vi "Create Message Setter (from Accessor).vi"(8 "error in (no error)":errorcluster, 10 "RPC Message Name":string, 11 "RPC Messages Folder (ProjectItem) in":refnum<vi>) -> (0 "error out":errorcluster, 1 "Created ?":bool, 2 "Getter VI out":refnum<vi>, 3 "RPC Messages Folder (ProjectItem) out":refnum<vi>)   [LabVIEW 2019, in "gRPC Template Creation Utility.lvlib"]
uses:
  gRPC Template Creation Utility.lvlib
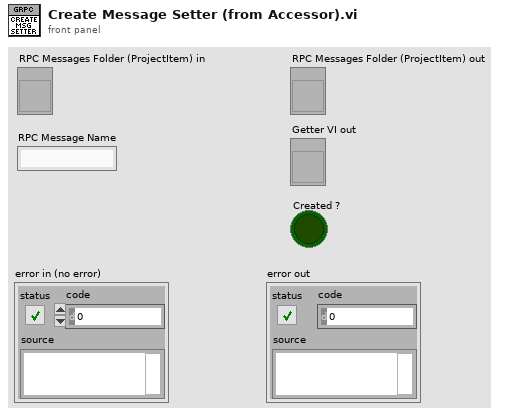
[diagram p1: front panel]
types:
  T1 = enum32{"invalid VI type", "Standard VI", "Control VI", "Global VI", "Polymorphic VI", "Configuration VI", "SubSystem", "Facade VI", "Method VI"}
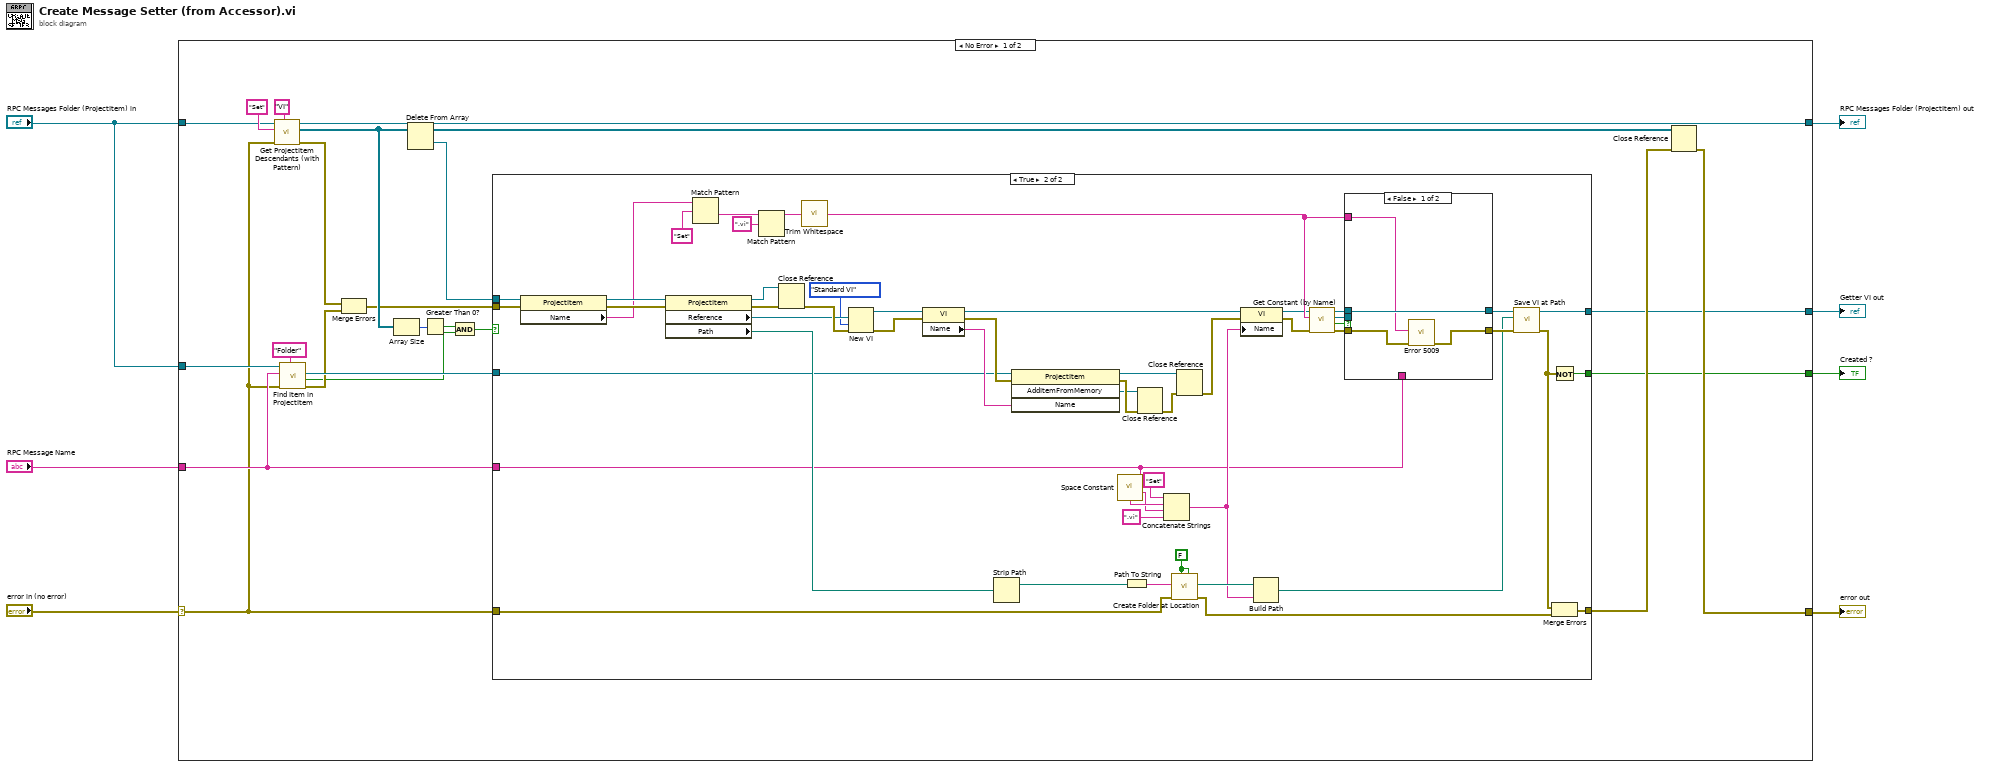
[diagram p0: block diagram]
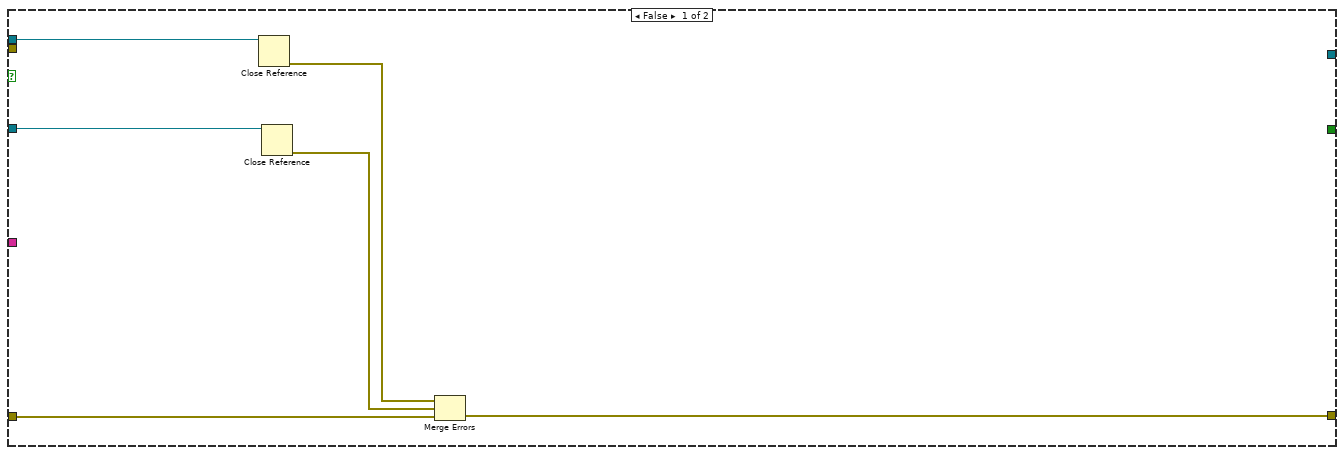
[diagram p2: hidden frame]
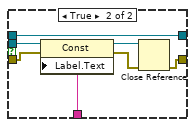
[diagram p3: hidden frame]
diagram:
  n1 = case shown="No Error" "error in (no error)" {
    selector: "error in (no error)" -> [w13 w100]
    tunnel: "RPC Message Name" -> [w25 _]
    tunnel: "RPC Messages Folder (ProjectItem) in" -> [w23 _]
    tunnel: "RPC Messages Folder (ProjectItem) in" -> [w18 w99]
    tunnel: [w11 w100] -> w4
    tunnel: [w10 w99] -> w3
    tunnel: [w9 _] -> w2
    tunnel: [w8 _] -> w1
    frame No Error {
      n2 = call "Get ProjectItem Descendants (with Pattern).vi"("Type"="VI", "error in (no error)"=w13, "Pattern"="Set", "ProjectItem in"=w18) -> ("error out"=w17:errorcluster, "ProjectItem descendents"=w24:refnum<vi>[], "ProjectItem out"=w10:refnum<vi>)  [unwired: 5 in]
      n3 = call "Find Item in ProjectItem.vi"("Item Type"="Folder", "error in (no error)"=w13, "Name"=w25, "ProjectItem in"=w23) -> ("error out"=w16:errorcluster, "Found ?"=w15:bool, "Item Refnum out"=w21:refnum<vi>)  [unwired: 4 in, 1 out]
      n4 = Merge Errors(w17, w16) -> (w14:errorcluster)
      n5 = Array Size(array=w24) -> (size(s)=w22:i32)
      n6 = Delete From Array(array=w24) -> (deleted portion=w27:refnum<vi>, array with subset deleted=w30:refnum<vi>[])  [unwired: 2 in]
      n7 = Greater Than 0?(x=w22) -> (x > 0?=w20:bool)
      n8 = And(x=w20, y=w15) -> (x .and. y?=w19:bool)
      n9 = case shown="True" w19 {
        tunnel: w25 -> [_ w38]
        tunnel: [w33 w84] -> w12
        tunnel: [_ w45] -> w8
        tunnel: w27 -> [w36 w59]
        tunnel: [_ w69] -> w9
        tunnel: w21 -> [w31 w64]
        tunnel: w13 -> [w32 w63]
        tunnel: w14 -> [_ w58]
        frame False {
          n10 = Close Reference(reference=w36) -> (error out=w34:errorcluster)  [unwired: 1 in]
          n11 = Close Reference(reference=w31) -> (error out=w35:errorcluster)  [unwired: 1 in]
          n12 = Merge Errors(w34, w35, w32) -> (w33:errorcluster)
        }
        frame True {
          w82 = FALSE ("Use Relative (F)")
          n13 = property class="ProjectItem"(reference=w59, error in=w58) -> (reference out=w57:refnum<vi>, error out=w56:errorcluster, "Name"=w55:string)
          n14 = property class="ProjectItem"(reference=w57, error in=w56) -> (reference out=w87:refnum<vi>, error out=w85:errorcluster, "Reference"=w75:refnum<vi>, "Path"=w78:path)
          n15 = Match Pattern(string=w55, regular expression="Set") -> (after substring=w53:string)  [unwired: 1 in, 3 out]
          n16 = Match Pattern(string=w53, regular expression=".vi") -> (before substring=w42:string)  [unwired: 1 in, 3 out]
          n17 = Close Reference(reference=w87, error in (no error)=w85) -> (error out=w86:errorcluster)
          n18 = call <vilib>:"Trim Whitespace.vi"("string"=w42) -> ("trimmed string"=w51:string)  [unwired: 1 in]
          n19 = New VI(8:w86, 9:T1."Standard VI" ("vi type (standard vi)"), 10:w75) -> (0:w74:errorcluster, 3:w72:refnum<vi>)  [unwired: 1 in, 3 out]
          n20 = property class="VI"(reference=w72, error in=w74) -> (reference out=w79:refnum<vi>, error out=w80:errorcluster, "Name"=w76:string)
          n21 = Strip Path(path=w78) -> (stripped path=w37:path)  [unwired: 1 out]
          n22 = invoke class="ProjectItem" method="AddItemFromMemory"(reference=w64, error in=w80, "Name"=w76) -> (reference out=w71:refnum<vi>, error out=w62:errorcluster, "AddItemFromMemory"=w61:refnum<vi>)  [unwired: 1 in, 1 out]
          n23 = call <vilib>:"Space Constant.vi"() -> ("String"=w67:string)
          n24 = Path To String(path=w37) -> (string=w77:string)
          n25 = Close Reference(reference=w61, error in (no error)=w62) -> (error out=w60:errorcluster)
          n26 = Concatenate Strings("Set" ("string"), w67, w38, ".vi" ("string")) -> (w65:string)
          n27 = call "Create Folder at Location.vi"("Override existing (F)"=w82, "Use Relative (F)"=w82, "Error In"=w63, "Path"=w77) -> ("Error Out"=w83:errorcluster, "Full path out"=w81:path)  [unwired: 5 in, 1 out]
          n28 = Close Reference(reference=w71, error in (no error)=w60) -> (error out=w70:errorcluster)
          n29 = property class="VI"(reference=w79, error in=w70, "Name"=w65) -> (reference out=w49:refnum<vi>, error out=w48:errorcluster)
          n30 = Build Path(base path=w81, name or relative path=w65) -> (appended path=w44:path)
          n31 = call "Get Constant (by Name).vi"("error in (no error)"=w48, "Constant Label"=w51, "Owner VI in"=w49) -> ("error out"=w47:errorcluster, "Found ?"=w41:bool, "Const ref out"=w50:refnum<vi>, "Owner VI out"=w40:refnum<vi>)  [unwired: 5 in]
          n32 = case shown="False" w41 {
            tunnel: w50 -> [_ w98]
            tunnel: w38 -> [_ w97]
            tunnel: w47 -> [w90 w96]
            tunnel: [w89 w93] -> w46
            tunnel: w40 -> [w91 w92]
            tunnel: [w91 w92] -> w39
            tunnel: w51 -> [w88 _]
            frame False {
              n33 = call "Error 5009.vi"("error in (no error)"=w90, "Cluster Definition Constant"=w88) -> ("error out"=w89:errorcluster)  [unwired: 9 in]
            }
            frame True {
              n34 = property class="Const"(reference=w98, error in=w96, "Label.Text"=w97) -> (reference out=w95:refnum<vi>, error out=w94:errorcluster)
              n35 = Close Reference(reference=w95, error in (no error)=w94) -> (error out=w93:errorcluster)
            }
          }
          n36 = call "Save VI at Path.vi"("error in (no error)"=w46, "Path"=w44, "VI in"=w39) -> ("error out"=w43:errorcluster, "VI out"=w45:refnum<vi>)  [unwired: 6 in, 1 out]
          n37 = Not(x=w43) -> (.not. x?=w69:bool)
          n38 = Merge Errors(w43, w83) -> (w84:errorcluster)
        }
      }
      n39 = Close Reference(reference=w30, error in (no error)=w12) -> (error out=w11:errorcluster)
    }
    frame Error {
    }
  }
  "error out" <- w4
  "RPC Messages Folder (ProjectItem) out" <- w3
  "Created ?" <- w2
  "Getter VI out" <- w1
